vi "Add Bitfile.vi"(8 "error in (no error)":errorcluster, 10 "Engine Simulation Toolkit Bitfile":T1, 11 "EST Custom Device in":refnum<k24>) -> (0 "error out":errorcluster, 3 "EST Custom Device out":refnum<k24>)   [LabVIEW 2015, in "Engine Simulation Toolkit Scripting API.lvlib"]
uses:
  Engine Simulation Toolkit Scripting API.lvlib
  NationalInstruments.VeriStand.SystemDefinitionAPI
  Bitfile.ctl
  Shared/Properties.vi
  <vilib>/NI Veristand/Custom Device API/Get Item Property (String Array).vi
  <vilib>/NI Veristand/Custom Device API/Set Item Property (String Array).vi
  <vilib>/NI Veristand/Custom Device API/Set Item Property (String).vi
  Shared/Engine Simulation Toolkit Shared.lvlib
  <vilib>/NI VeriStand/Custom Device API/Custom Device API.lvlib
  System Explorer/Engine Simulation Toolkit System Explorer.lvlib
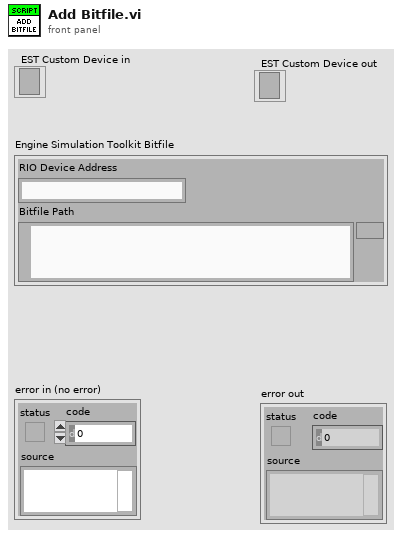
[diagram p1: front panel]
types:
  T1 = typedef "Engine Simulation Toolkit Scripting API.lvlib/Bitfile.ctl" = cluster{"RIO Device Address":string, "Bitfile Path":path}
  T2 = typedef "Custom Device API.lvlib/Custom Device Item Ref.ctl" = u64
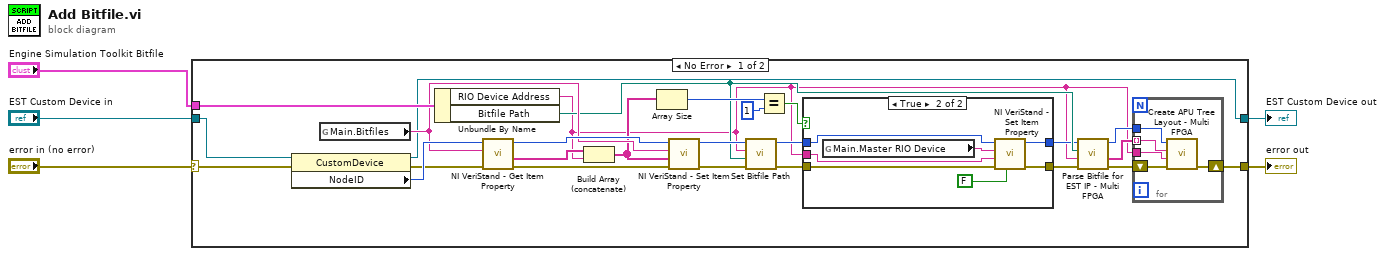
[diagram p0: block diagram]
diagram:
  n1 = case shown="No Error" "error in (no error)" {
    selector: "error in (no error)" -> [w29 w47]
    tunnel: [w7 w47] -> w5
    tunnel: "EST Custom Device in" -> [w30 w46]
    tunnel: [w6 w46] -> w2
    tunnel: "Engine Simulation Toolkit Bitfile" -> [w31 _]
    frame No Error {
      n2 = property class="CustomDevice"(reference=w30, error in=w29) -> (reference out=w6:refnum<k24>, error out=w24:errorcluster, "NodeID"=w27:u64)
      n3 = global read "Properties.vi" "Main.Bitfiles"() -> (w21:string)
      n4 = Unbundle By Name(w31) -> ("RIO Device Address"=w8:string, "Bitfile Path"=w13:path)
      n5 = call-poly <vilib>:"NI VeriStand - Get Item Property.vi"("error in (no error)"=w24, "Property Name"=w21, "Item Ref in"=w27) -> ("error out"=w25:errorcluster, "Value"=w28:string[], "Item Ref out"=w26:T2)  [unwired: 5 in, 1 out]
      n6 = Build Array (concatenate)(w28, w8) -> (w18:string[])
      n7 = Array Size(array=w18) -> (size(s)=w20:i32)
      n8 = call-poly <vilib>:"NI VeriStand - Set Item Property.vi"("error in (no error)"=w25, "Value"=w18, "Property Name"=w21, "Item Ref in"=w26) -> ("error out"=w22:errorcluster, "Item Ref out"=w23:T2)  [unwired: 5 in, 1 out]
      n9 = call "Set Bitfile Path.vi"("error in (no error)"=w22, "Bitfile Path in"=w13, "RIO Device Address in"=w8, "Item Ref in"=w23) -> ("error out"=w16:errorcluster, "Item Ref out"=w15:T2)  [unwired: 6 in]
      n10 = Equal?(x=w20, y=1) -> (x = y?=w17:bool)
      n11 = case shown="True" w17 {
        tunnel: w16 -> [w37 w44]
        tunnel: [w37 w43] -> w11
        tunnel: w15 -> [w38 w42]
        tunnel: w8 -> [_ w41]
        tunnel: [w38 w40] -> w12
        frame False {
        }
        frame True {
          n12 = global read "Properties.vi" "Main.Master RIO Device"() -> (w45:string)
          n13 = call-poly <vilib>:"NI VeriStand - Set Item Property.vi"("Binary String (T)"=FALSE, "error in (no error)"=w44, "Value"=w41, "Property Name"=w45, "Item Ref in"=w42) -> ("error out"=w43:errorcluster, "Item Ref out"=w40:T2)  [unwired: 4 in, 1 out]
        }
      }
      n14 = call "Parse Bitfile for EST IP - Multi FPGA.vi"("error in (no error)"=w11, "RIO device address"=w8, "bitfile path"=w13, "Item Ref in"=w12) -> ("error out"=w10:errorcluster, "APUs"=w14:string[], "Item Ref out"=w9:T2)  [unwired: 4 in, 1 out]
      n15 = for {
        shift-right: [w35] -> w7
        shift-left: w10 -> [w36]
        tunnel: w14 -> [w33] mode=indexing
        tunnel: w8 -> [w32]
        tunnel: w9 -> [w34]
        n16 = call "Create APU Tree Layout - Multi FPGA.vi"("error in (no error)"=w36, "rio name"=w32, "engine name"=w33, "Section Ptr"=w34) -> ("error out"=w35:errorcluster)  [unwired: 5 in, 2 out]
      }
    }
    frame Error {
    }
  }
  "EST Custom Device out" <- w2
  "error out" <- w5
